vi "ScanPlot.vi"(8 "error in":errorcluster, 11 "variant in":variant) -> (0 "error out":errorcluster, 1 "3rd Dim":u32, 2 "2nd Dim":u32, 3 "variant out":variant, 4 "Intensity Graph":dbl[][](graph), 6 "XY Graph":T1(graph))   [LabVIEW 2013]
uses:
  <vilib>/Analysis/1siggen.llb/Ramp Pattern by Samples.vi
  <vilib>/Analysis/NI_AALBase.lvlib
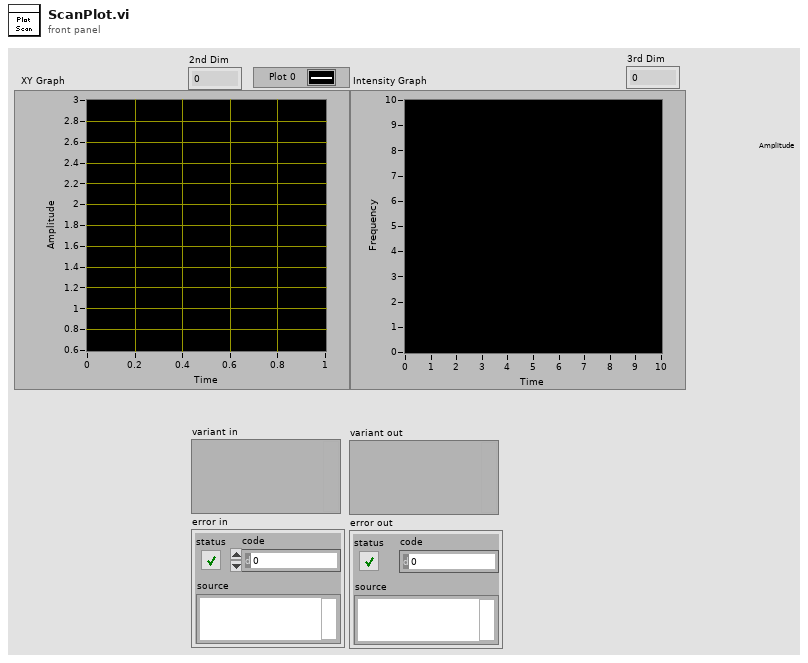
[diagram p1: front panel]
types:
  T1 = cluster{"Ramp Pattern":dbl[], "Ramp Pattern":dbl[]}
  T2 = cluster{"Ramp Pattern":dbl[], "initialized array":dbl[]}
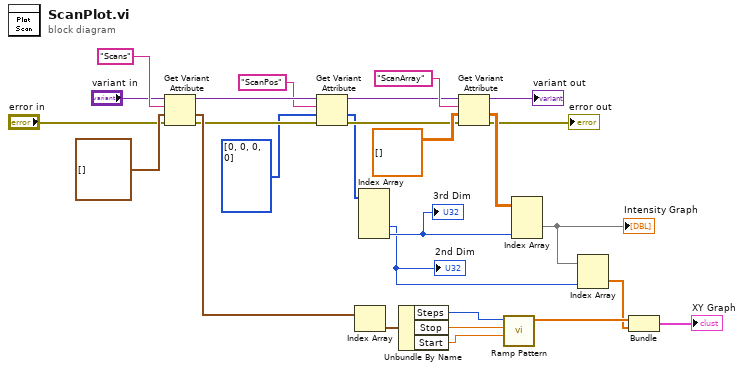
[diagram p0: block diagram]
diagram:
  n1 = Get Variant Attribute(Variant="variant in", name="Scans", default value (empty Variant)=cluster{"Start":dbl, "Stop":dbl, "Steps":u32}[] [], error in="error in") -> (duplicate Variant=w16:variant, value=w20:cluster{"Start":dbl, "Stop":dbl, "Steps":u32}[], error out=w17:errorcluster)  [unwired: 1 out]
  n2 = Get Variant Attribute(Variant=w16, name="ScanPos", default value (empty Variant)=i32[] [0, 0, 0, 0], error in=w17) -> (duplicate Variant=w6:variant, value=w5:i32[], error out=w7:errorcluster)  [unwired: 1 out]
  n3 = Index Array(array=w20) -> (element=w21:cluster{"Start":dbl, "Stop":dbl, "Steps":u32})  [unwired: 1 in]
  n4 = Index Array(array=w5) -> (element #3=w1:i32, element #4=w2:i32)  [unwired: 4 in, 2 out]
  "3rd Dim" <- w2
  "2nd Dim" <- w1
  n5 = Unbundle By Name(w21) -> ("Steps"=w22:u32, "Stop"=w23:dbl, "Start"=w24:dbl)
  n6 = Get Variant Attribute(Variant=w6, name="ScanArray", default value (empty Variant)=dbl[][][] [] ("initialized array"), error in=w7) -> (duplicate Variant=→"variant out":variant, value=w12:dbl[][][], error out=→"error out":errorcluster)  [unwired: 1 out]
  n7 = call-poly <vilib>:"Ramp Pattern.vi"("start"=w24, "end"=w23, "samples"=w22) -> ("Ramp Pattern"=w27:dbl[])  [unwired: 7 in, 1 out]
  n8 = Index Array(array=w12, index (dim 2)=w2) -> (element=w13:dbl[][])  [unwired: 2 in]
  "Intensity Graph" <- w13
  n9 = Index Array(array=w13, index (col)=w1) -> (element=w26:dbl[])  [unwired: 1 in]
  n10 = Bundle("Ramp Pattern"=w27, "initialized array"=w26) -> (→"XY Graph":T2)  [unwired: 1 in]
